vi "Measure - NI 9215.vi"(8 "Error In":errorcluster) -> (0 "Error Out":errorcluster)   [LabVIEW 2011]
uses:
  <vilib>/DAQmx/read.llb/DAQmx Read.vi
  <vilib>/DAQmx/read.llb/DAQmx Read (Analog 1D Wfm NChan NSamp).vi
  <vilib>/DAQmx/miscellaneous.llb/DAQmx Fill In Error Info.vi
panel:
  out "data":waveform(dbl)[](graph) caption="Chart"
  in  "stop":bool
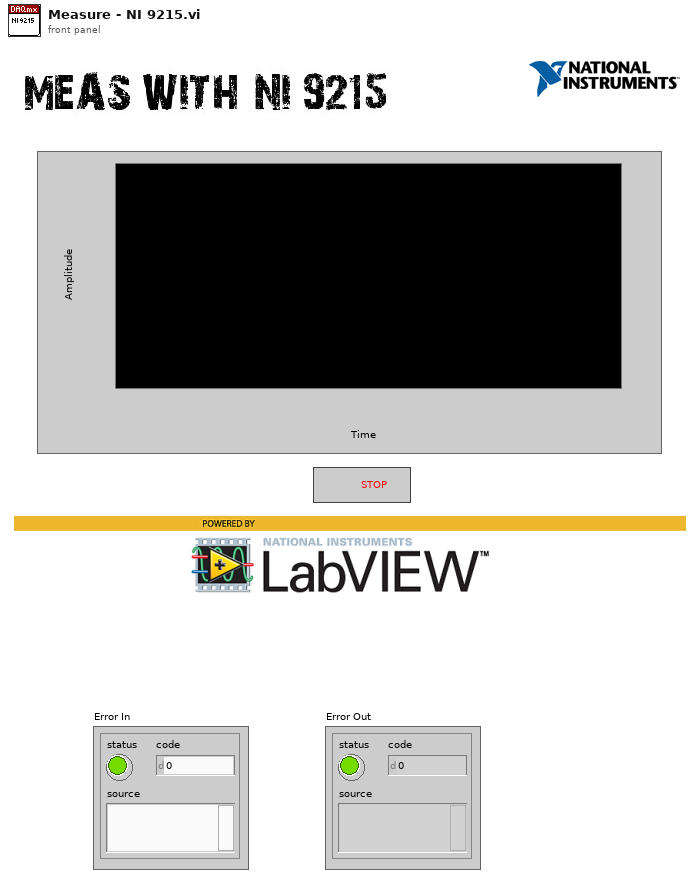
[diagram p1: front panel]
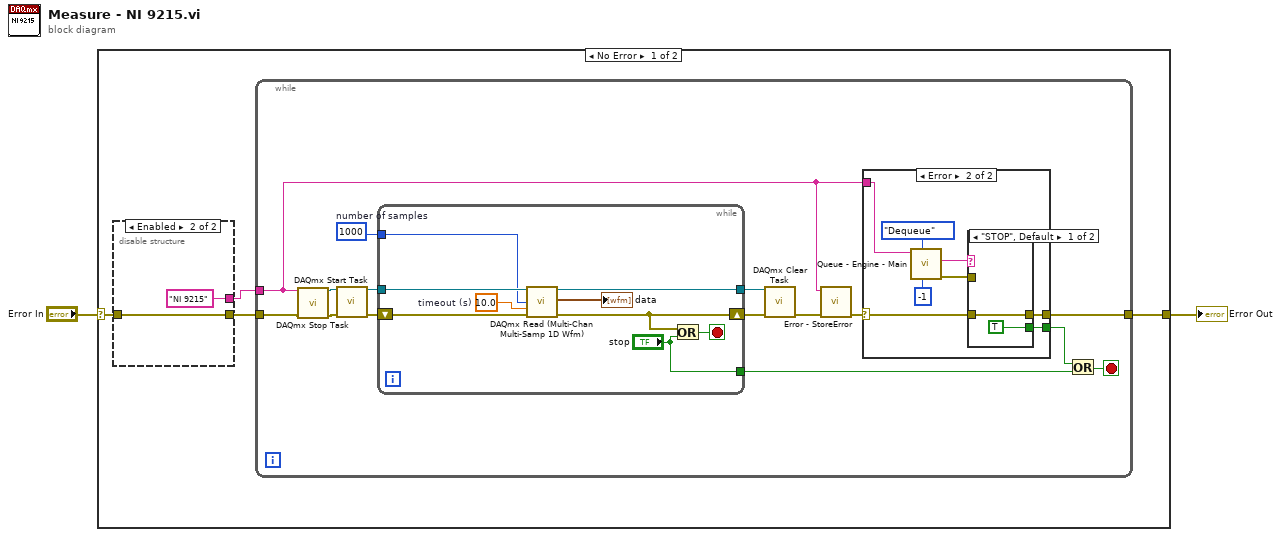
[diagram p0: block diagram]
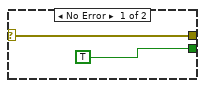
[diagram p2: hidden frame]
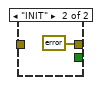
[diagram p3: hidden frame]
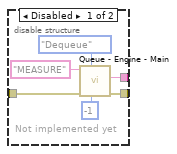
[diagram p4: hidden frame]
diagram:
  n1 = case shown="No Error" "Error In" {
    selector: "Error In" -> [w6 w52]
    tunnel: [w5 w52] -> w2
    frame No Error {
      n2 = disable-structure shown="Enabled" {
        disable-tunnel: [w46 w51] -> w3
        disable-tunnel: [w45 "NI 9215" ("Variable In")] -> w4
        disable-tunnel: w6 -> [w44 w51]
        frame Disabled {
          # "Not implemented yet"
          n3 = call "Queue - Engine - Main.vi"("timeout in ms (-1)"=-1, "Operation"=enum16{"Enqueue", "Dequeue", "Flush", "Release"}."Dequeue", "error in"=w44, "Queue Name In"="MEASURE") -> ("error out"=w46:errorcluster, "Data Out"=w45:string)  [unwired: 5 in, 1 out]
        }
        frame Enabled {
        }
      }
      n4 = while {
        tunnel: [w11] -> w5
        tunnel: w4 -> [w7]
        tunnel: w3 -> [w13]
        stop <- w8 stop-if-true
        w19 = 1000  # number of samples
        n5 = call <vilib>:"DAQmx Stop Task.vi"("task/channels in"=w7, "error in"=w13) -> ("task out"=w16:refnum<k21>, "error out"=w15:errorcluster)  [unwired: 12 in]
        n6 = call <vilib>:"DAQmx Start Task.vi"("task/channels in"=w16, "error in"=w15) -> ("task out"=w21:refnum<k21>, "error out"=w20:errorcluster)  [unwired: 12 out]
        n7 = while {
          tunnel: w21 -> [w43]
          tunnel: w19 -> [w39]
          tunnel: [w40] -> w17
          shift-right: [w37] -> w18
          shift-left: w20 -> [w42]
          tunnel: ["stop"] -> w9
          stop <- w38 stop-if-true
          w36 = 10.0  # timeout (s)
          n8 = call-poly "DAQmx Read (Multi-Chan Multi-Samp 1D Wfm).vi"("task/channels in"=w43, "number of samples per channel"=w39, "timeout"=w36, "error in"=w42) -> ("task out"=w40:refnum<k21>, "data"=→"data":waveform(dbl)[], "error out"=w37:errorcluster)  [unwired: 9 out]
          n9 = Or(x=w37, y="stop") -> (x .or. y?=w38:bool)
        }
        n10 = call <vilib>:"DAQmx Clear Task.vi"("task in"=w17, "error in"=w18) -> ("error out"=w14:errorcluster)  [unwired: 13 out]
        n11 = call "Error - StoreError.vi"("Error In"=w14, "Error Source In"=w7) -> ("Error Out"=w12:errorcluster)  [unwired: 8 in, 1 out]
        n12 = case shown="Error" w12 {
          selector: w12 -> [w23 w24]
          tunnel: [w23 w26] -> w11
          tunnel: [TRUE w25] -> w10
          tunnel: w7 -> [_ w29]
          frame No Error {
          }
          frame Error {
            n13 = call "Queue - Engine - Main.vi"("timeout in ms (-1)"=-1, "Operation"=enum16{"Enqueue", "Dequeue", "Flush", "Release"}."Dequeue", "Queue Name In"=w29) -> ("error out"=w28:errorcluster, "Data Out"=w27:string)  [unwired: 6 in, 1 out]
            n14 = case shown="\"STOP\", Default" w27 {
              tunnel: w28 -> [_ _]
              tunnel: [w32 errorcluster {"status"=FALSE, "code"=0, "source"=""} ("error out")] -> w26
              tunnel: [TRUE _] -> w25
              tunnel: w24 -> [w32 _]
              frame "STOP", Default {
              }
              frame "INIT" {
              }
            }
          }
        }
        n15 = Or(x=w10, y=w9) -> (x .or. y?=w8:bool)
      }
    }
    frame Error {
    }
  }
  "Error Out" <- w2
